vi "Pull SR Data.vi"(8 "error in (no error)":errorcluster, 11 "number":i32) -> (0 "error out":errorcluster, 2 "SR Cluster out":T1 {"Creation Date" format="%<%x>T"; "Last Updated" format="%<%x>T"}, 3 "SR Notes array":T3[](array[typedef]) {"Note Date" format="%<%x >T"})   [LabVIEW 2018]
uses:
  Type Defs/SR Note Cluster.ctl
  Type Defs/SR Cluster.ctl
  Type Defs/SR Status.ctl
  <vilib>/httpClient/LabVIEWHTTPClient.lvlib
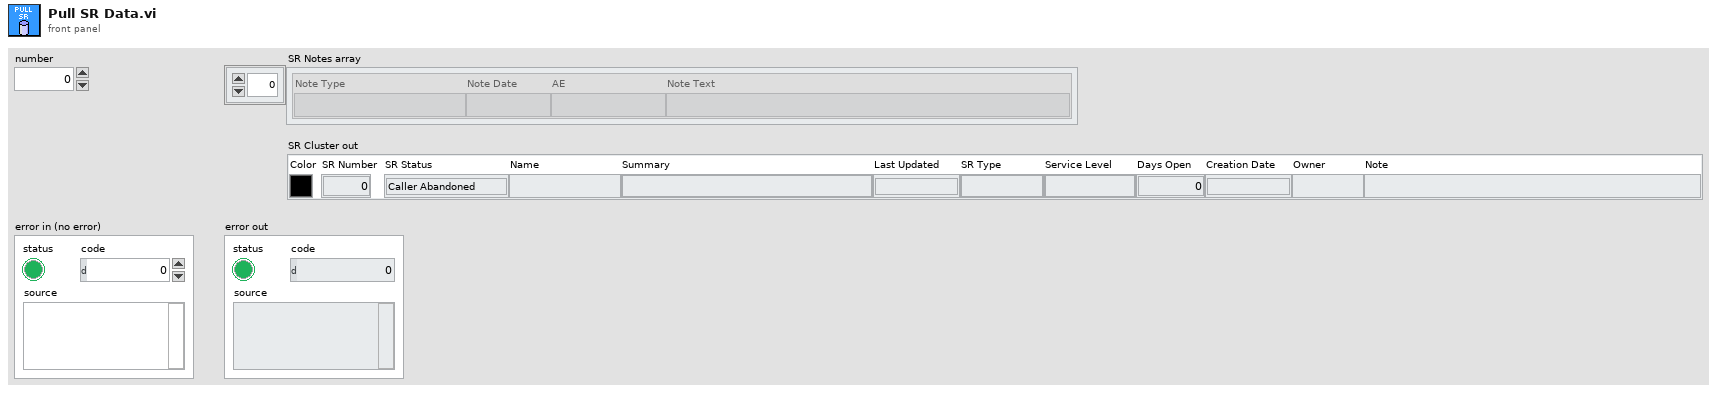
[diagram p1: front panel]
types:
  T1 = typedef "SR Cluster.ctl" = cluster{"Color":u32, "SR Number":i32, "SR Status":T2, "Name":string, "Summary":string, "Last Updated":timestamp, "SR Type":string, "Service Level":string, "Days Open":dbl, "Creation Date":timestamp, "Owner":string, "Note":string}
  T2 = typedef "SR Status.ctl" = enum16{"Caller Abandoned", "Created in Error", "Expired", "Forum Resolved AE", "Forum Resolved Customer", "IN WORK", "IN WORK Collab with AES", "IN WORK Collab with PSE", "IN WORK Collab with SE", "IN WORK Customer Added Note", "IN WORK Escalation", "IN WORK Wait on Customer", "Open", "Potentially Resolved", "Presumed Resolved", "RMA Approved for Return", "RMA Closed", "RMA Closed - DOA", "RMA In Progress", "RMA Open", "RMA Waiting on Customer", "Resolved", "Passed Off"}
  T3 = typedef "SR Note Cluster.ctl" = cluster{"Note Type":string, "Note Date":timestamp, "AE":string, "Note Text":string}
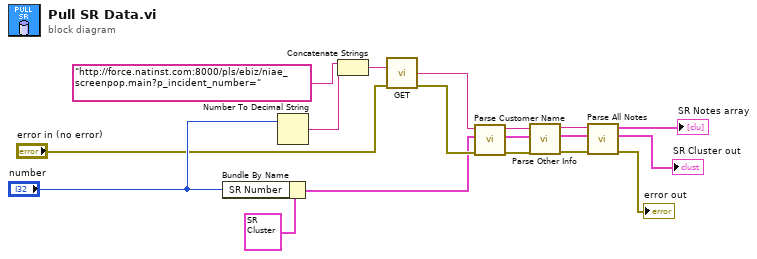
[diagram p0: block diagram]
diagram:
  n1 = Bundle By Name(cluster=T1 {"Color"=0, "SR Number"=0, "SR Status"=enum."Caller Abandoned", "Name"="", "Summary"="", "Last Updated"=timestamp(0 s since 1904-01-01), "SR Type"="", "Service Level"="", "Days Open"=0.0, "Creation Date"=timestamp(0 s since 1904-01-01), "Owner"="", "Note"=""} ("SR Cluster"), "SR Number"="number") -> (w9:T1)
  n2 = Number To Decimal String(number="number") -> (decimal integer string=w2:string)  [unwired: 1 in]
  n3 = Concatenate Strings("http://force.natinst.com:8000/pls/ebiz/niae_screenpop.main?p_incident_number=" ("string"), w2) -> (w3:string)
  n4 = call <vilib>:"GET.vi"("url"=w3, "error in (no error)"="error in (no error)") -> ("body"=w8:string, "error out"=w15:errorcluster)  [unwired: 10 in, 2 out]
  n5 = call "Parse Customer Name.vi"("error in"=w15, "SR Cluster in"=w9, "HTML text in"=w8) -> ("error out"=w16:errorcluster, "SR Cluster out"=w10:T1, "remaining string out"=w11:string)  [unwired: 6 in]
  n6 = call "Parse Other Info.vi"("error in (no error)"=w16, "SR Cluster in"=w10, "remaining string in"=w11) -> ("error out"=w14:errorcluster, "SR Cluster out"=w13:T1, "result string"=w12:string)  [unwired: 6 in]
  n7 = call "Parse All Notes.vi"("error in (no error)"=w14, "SR Cluster in"=w13, "result string"=w12) -> ("error out"=→"error out":errorcluster, "SR Cluster out"=→"SR Cluster out":T1, "SR Notes array"=→"SR Notes array":T3[])  [unwired: 6 in]
